vi "Generate Staircase Waveforms.vi"(6 "sampling info":cluster{"Fs":dbl, "#s":dbl}={"Fs"=1000.0, "#s"=1000.0} {"Fs" format="%.2p"}, 8 "error in (no error)":errorcluster, 9 "reset?":bool, 10 "updates before reset":i32=10, 11 "Generator in":refnum<class "Generator.lvclass">) -> (0 "error out":errorcluster, 2 "waveform out":waveform(dbl), 3 "Generator out":refnum<class "Generator.lvclass">)   [LabVIEW 2019, in "Generator.lvclass"]
uses:
  Generator.lvclass
  <vilib>/Analysis/1siggen.llb/Ramp Pattern by Samples.vi
  <vilib>/Analysis/NI_AALBase.lvlib
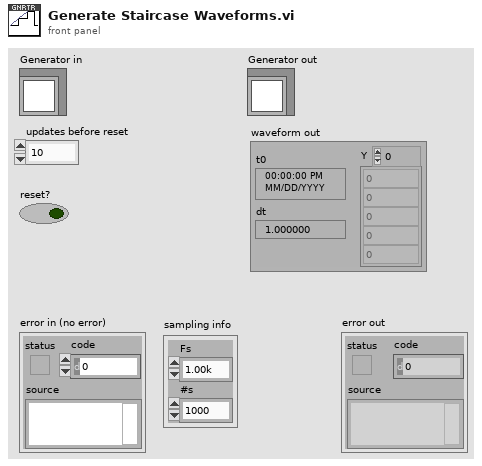
[diagram p1: front panel]
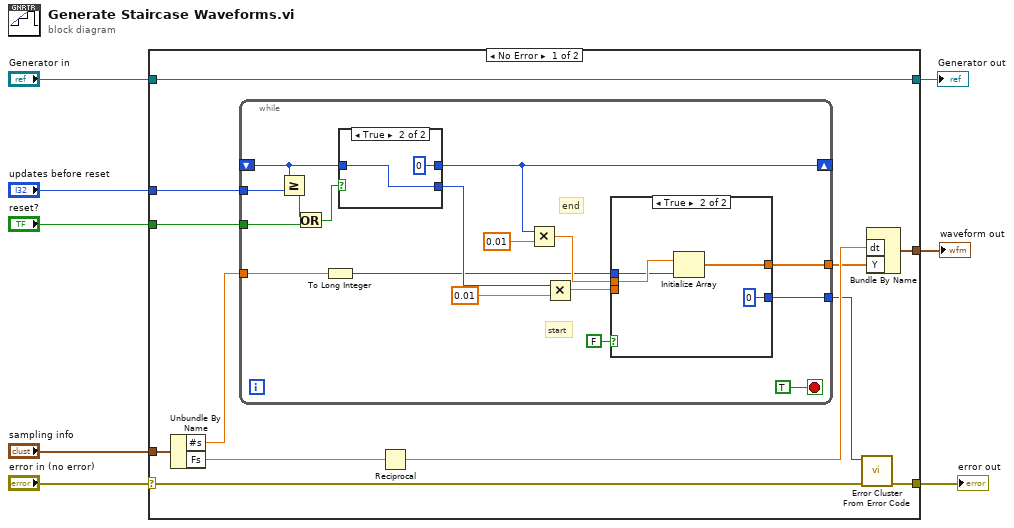
[diagram p0: block diagram]
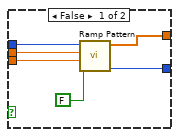
[diagram p2: hidden frame]
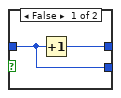
[diagram p3: hidden frame]
diagram:
  n1 = case shown="No Error" "error in (no error)" {
    selector: "error in (no error)" -> [w10 w53]
    tunnel: "updates before reset" -> [w20 _]
    tunnel: "reset?" -> [w19 _]
    tunnel: "sampling info" -> [w18 _]
    tunnel: [w14 _] -> w5
    tunnel: [w11 w53] -> w4
    tunnel: [w9 w52] -> w2
    tunnel: "Generator in" -> [w9 w52]
    frame No Error {
      n2 = Unbundle By Name(w18) -> ("#s"=w17:dbl, "Fs"=w16:dbl)
      n3 = while {
        shift-right: [w27] -> _
        shift-left: _ -> [w35]
        tunnel: [w23] -> w13
        tunnel: w17 -> [w34]
        tunnel: w20 -> [w33]
        tunnel: w19 -> [w32]
        tunnel: [w22] -> w12
        stop <- TRUE stop-if-true
        # "end"
        # "start"
        n4 = Greater Or Equal?(x=w35, y=w33) -> (x >= y?=w31:bool)
        n5 = Or(x=w31, y=w32) -> (x .or. y?=w30:bool)
        n6 = To Long Integer(number=w34) -> (32bit integer=w21:i32)
        n7 = case shown="True" w30 {
          tunnel: [w49 0] -> w27
          tunnel: w35 -> [w48 w50]
          tunnel: [w48 w50] -> w25
          frame False {
            n8 = Increment(x=w48) -> (x+1=w49:i32)
          }
          frame True {
          }
        }
        n9 = Multiply(x=w27, y=0.01 ("x")) -> (x*y=w28:dbl)
        n10 = Multiply(x=w25, y=0.01 ("x")) -> (x*y=w24:dbl)
        n11 = case shown="True" FALSE {
          tunnel: w28 -> [w41 w47]
          tunnel: [w43 w46] -> w23
          tunnel: w21 -> [w42 w45]
          tunnel: w24 -> [w40 _]
          tunnel: [w38 0 ("error")] -> w22
          frame False {
            n12 = call-poly <vilib>:"Ramp Pattern.vi"("exclude end?"=FALSE, "start"=w40, "end"=w41, "samples"=w42) -> ("error"=w38:i32, "Ramp Pattern"=w43:dbl[])  [unwired: 6 in]
          }
          frame True {
            n13 = Initialize Array(w47, w45) -> (w46:dbl[])
          }
        }
      }
      n14 = Reciprocal(x=w16) -> (1/x=w15:dbl)
      n15 = call <vilib>:"Error Cluster From Error Code.vi"("error in (no error)"=w10, "error code (0)"=w12) -> ("error out"=w11:errorcluster)  [unwired: 7 in]
      n16 = Bundle By Name("dt"=w15, "Y"=w13) -> (w14:waveform(dbl))  [unwired: 1 in]
    }
    frame Error {
    }
  }
  "waveform out" <- w5
  "error out" <- w4
  "Generator out" <- w2
